vi "UIRef.vi"(8 "error in":errorcluster, 11 "EthernetIP editor node in":refnum<class "EthernetIP editor node.lvclass">) -> (0 "error out":errorcluster, 2 "VI refnum":refnum<vi>, 3 "EthernetIP editor node out":refnum<class "EthernetIP editor node.lvclass">)   [LabVIEW 2013, in "EthernetIP editor node.lvclass"]
uses:
  EthernetIP editor node.lvclass
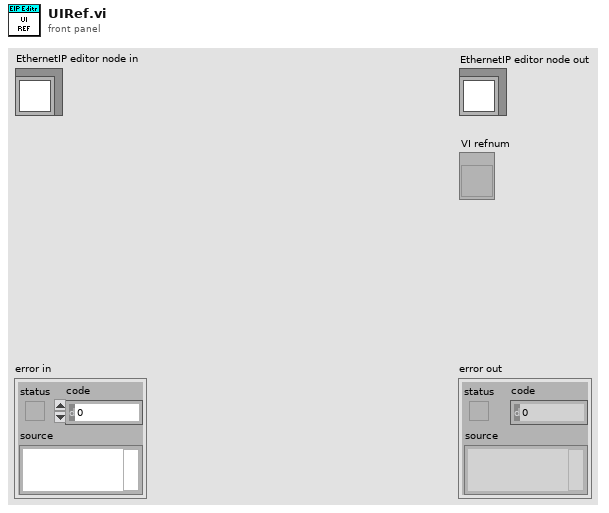
[diagram p1: front panel]
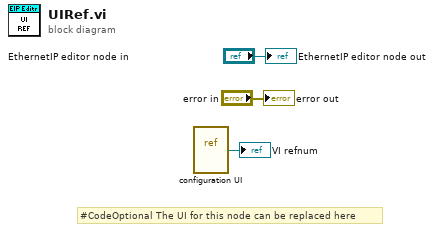
[diagram p0: block diagram]
diagram:
  # "#CodeOptional The UI for this node can be replaced here"
  n1 = vi-ref "configuration UI.vi"() -> (→"VI refnum":refnum<vi>)
  "error out" <- "error in"
  "EthernetIP editor node out" <- "EthernetIP editor node in"
